vi "DFD Get Lattice Coef.vi"(7 "type (FLP)":enum16{"FLP", "FXP"}(ring), 8 "error in (no error)":errorcluster, 11 "filter in":T2={"mSRate_Fs"=1.0, "mSRate_Version"="2.0", "mSRate_Comments"="", "mSRate_OrgCoef"={"type"=enum."Undefined", "gain"=1.0, "coef a (k)"=[], "coef b (v)"=[]}, "mSRate_CurCoef"={"type"=enum."Undefined", "gain"=1.0, "coef a (k)"=[], "coef b (v)"=[]}, "mSRate_Quantized?"=FALSE, "mSRate_QCoef"={"type"=enum."Undefined", "gain"=1.0, "coef a (k)"=[], "coef b (v)"=[]}, "mSRate_QSettings"=[], "mSRate_Order"=0, "mSRate_Scaling"={"mSRate_ScaleByPowerOf2?"=FALSE, "mSRate_ScaleType"=enum."No Norm"}} {"mSRate_QSettings"."source" items=["Coef a/k"=0, "Coef b/v"=7, "Input"=1, "Output"=2, "Multiplicand"=3, "Product"=4, "Sum"=5, "Delay"=6, "Gain"=8]}) -> (0 "error out":errorcluster, 2 "lattice coef":T1 {"structure type" items=["Invalid"=0, "Lattice Allpass (basic sections)"=13, "Lattice Allpass (one multiplier sections)"=14, "Lattice Allpass (normalized sections)"=15, "Lattice AR (basic sections)"=16, "Lattice AR (one multiplier sections)"=17, "Lattice AR (normalized sections)"=18, "Lattice MA (minimum phase)"=19, "Lattice MA (maximum phase)"=20, "Lattice ARMA (basic sections)"=21, "Lattice ARMA (one multiplier sections)"=22, "Lattice ARMA (normalized sections)"=23]}, 3 "filter out":T2={"mSRate_Fs"=1.0, "mSRate_Version"="2.0", "mSRate_Comments"="", "mSRate_OrgCoef"={"type"=enum."Undefined", "gain"=1.0, "coef a (k)"=[], "coef b (v)"=[]}, "mSRate_CurCoef"={"type"=enum."Undefined", "gain"=1.0, "coef a (k)"=[], "coef b (v)"=[]}, "mSRate_Quantized?"=FALSE, "mSRate_QCoef"={"type"=enum."Undefined", "gain"=1.0, "coef a (k)"=[], "coef b (v)"=[]}, "mSRate_QSettings"=[], "mSRate_Order"=0, "mSRate_Scaling"={"mSRate_ScaleByPowerOf2?"=FALSE, "mSRate_ScaleType"=enum."No Norm"}} {"mSRate_QSettings"."source" items=["Coef a/k"=0, "Coef b/v"=7, "Input"=1, "Output"=2, "Multiplicand"=3, "Product"=4, "Sum"=5, "Delay"=6, "Gain"=8]})   [LabVIEW 2017, in "NI_DigFilterLicensed.lvlib"]
doc: "Retrieves the lattice form coefficients of a filter. The filter you specify must have a lattice form filter structure."
uses:
  <vilib>/addons/Digital Filter Design/NI_DigFilterLicensed.lvlib
  <vilib>/addons/Digital Filter Design/_Objects.llb/DFD Filter Obj.ctl
  <vilib>/addons/Digital Filter Design/_Objects.llb/DFD Filter Coef.ctl
  <vilib>/addons/Digital Filter Design/_Objects.llb/DFD Filter Structure Type Selector.ctl
  <vilib>/addons/Digital Filter Design/_Objects.llb/dfd_Internal Quantization Settings.ctl
  <vilib>/addons/Digital Filter Design/_Objects.llb/dfd_Internal Quantization Srcs.ctl
  <vilib>/addons/Digital Filter Design/_Objects.llb/DFD Coef Norm Type.ctl
  <vilib>/addons/Digital Filter Design/_Objects.llb/DFD Filter Structure Form Id.ctl
  <vilib>/addons/Digital Filter Design/_Misc.llb/dfd_Error Cluster From Error Code (Scalar).vi
  <vilib>/addons/Digital Filter Design/FilterLib.llb/dfd_Get Filter Coef Type (Filter IO).vi
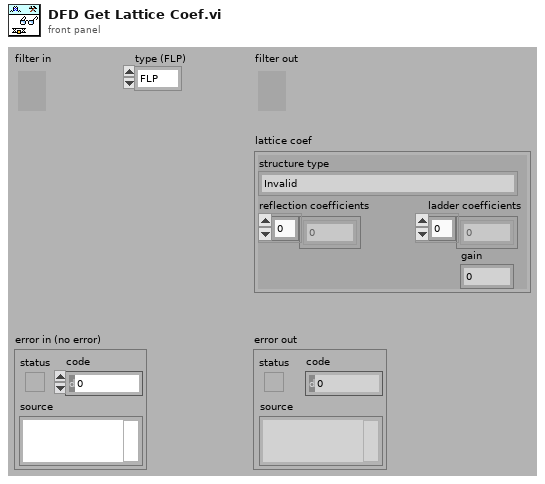
[diagram p1: front panel]
types:
  T1 = cluster{"structure type":u16, "reflection coefficients":dbl[], "ladder coefficients":dbl[], "gain":dbl}
  T2 = typedef "NI_DigFilterLicensed.lvlib/DFD Filter Obj.ctl" = cluster{"mSRate_Fs":dbl, "mSRate_Version":string, "mSRate_Comments":string, "mSRate_OrgCoef":T3, "mSRate_CurCoef":T3, "mSRate_Quantized?":bool, "mSRate_QCoef":T3, "mSRate_QSettings":T5[], "mSRate_Order":i32, "mSRate_Scaling":cluster{"mSRate_ScaleByPowerOf2?":bool, "mSRate_ScaleType":T7}}
  T3 = typedef "NI_DigFilterLicensed.lvlib/DFD Filter Coef.ctl" = cluster{"type":T4, "gain":dbl, "coef a (k)":dbl[], "coef b (v)":dbl[]}
  T4 = typedef "NI_DigFilterLicensed.lvlib/DFD Filter Structure Type Selector.ctl" = enum16{"Undefined", "FIR Direct Form", "FIR Direct Form Transposed", "FIR Symmetric", "FIR Antisymmetric", "IIR Direct Form I", "IIR Direct Form I Transposed", "IIR Direct Form II", "IIR Direct Form II Transposed", "IIR Cascaded Second Order Sections Form I", "IIR Cascaded Second Order Sections Form I Transposed", "IIR Cascaded Second Order Sections Form II", "IIR Cascaded Second Order Sections Form II Transposed", "Lattice Allpass (basic sections)", "Lattice Allpass (one multiplier sections)", "Lattice Allpass (normalized sections)", "Lattice AR (basic sections)", "Lattice AR (one multiplier sections)", "Lattice AR (normalized sections)", "Lattice MA (minimum phase)", "Lattice MA (maximum phase)", "Lattice ARMA (basic sections)", "Lattice ARMA (one multiplier sections)", "Lattice ARMA (normalized sections)"}
  T5 = typedef "NI_DigFilterLicensed.lvlib/dfd_Internal Quantization Settings.ctl" = cluster{"source":T6, "wl":i16, "iwl":i16, "overflow mode":enum16{"Saturation", "Wrap"}, "rounding mode":enum16{"Nearest", "Truncation"}, "signed?":bool}
  T6 = typedef "NI_DigFilterLicensed.lvlib/dfd_Internal Quantization Srcs.ctl" = u16
  T7 = typedef "NI_DigFilterLicensed.lvlib/DFD Coef Norm Type.ctl" = enum16{"No Norm", "Time Domain 1-Norm", "Time Domain 2-Norm", "Time Domain Inf-Norm"}
  T8 = typedef "NI_DigFilterLicensed.lvlib/DFD Filter Structure Form Id.ctl" = enum16{"Undefined", "Direct Form", "SOS Form", "Lattice Form"}
  T9 = cluster{"structure type":T4, "k":dbl[], "v":dbl[], "gain":dbl}
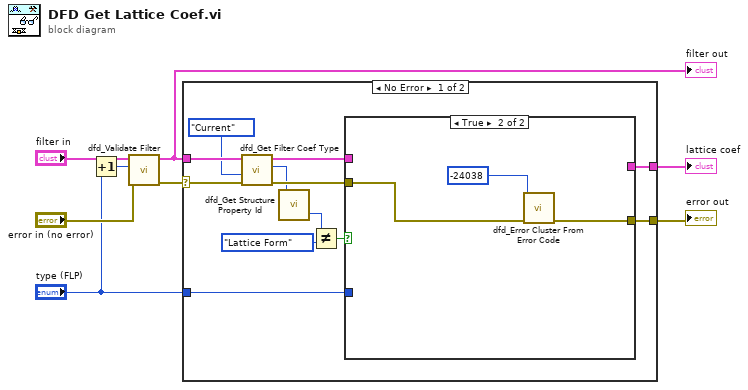
[diagram p0: block diagram]
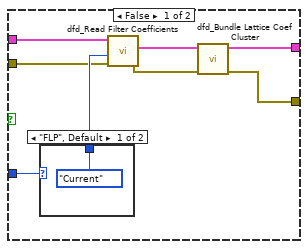
[diagram p2: hidden frame]
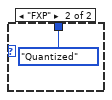
[diagram p3: hidden frame]
diagram:
  n1 = Increment(x="type (FLP)") -> (x+1=w2:enum16{"FLP", "FXP"})
  n2 = call <vilib>:"dfd_Validate Filter.vi"("error in (no error)"="error in (no error)", "check option"=w2, "filter in"="filter in") -> ("error out"=w3:errorcluster, "filter out"=w5:T2)  [unwired: 7 out]
  "filter out" <- w5
  n3 = case shown="No Error" w3 {
    selector: w3 -> [w12 w34]
    tunnel: [w16 w34] -> w8
    tunnel: w5 -> [w14 _]
    tunnel: [w17 _] -> w7
    tunnel: "type (FLP)" -> [w15 _]
    frame No Error {
      n4 = call-poly <vilib>:"dfd_Get Filter Coef Type.vi"("error in (no error)"=w12, "coef source"=enum16{"Original", "Current", "Quantized"}."Current", "filter in"=w14) -> ("error out"=w10:errorcluster, "type"=w9:T4, "filter out"=w13:T2)  [unwired: 1 in, 5 out]
      n5 = call <vilib>:"dfd_Get Structure Property Id.vi"("structure type"=w9) -> ("filter structure form id"=w19:T8)  [unwired: 1 out]
      n6 = Not Equal?(x=w19, y=DFD_Filter_Structure_Form_Id."Lattice Form" ("filter structure form id")) -> (x != y?=w18:bool)
      n7 = case shown="True" w18 {
        tunnel: w13 -> [w28 _]
        tunnel: [w25 _] -> w17
        tunnel: [w24 w32] -> w16
        tunnel: w15 -> [w23 _]
        tunnel: w10 -> [w21 w31]
        frame False {
          n8 = case shown="\"FLP\", Default" w23 {
            tunnel: [enum16{"Original", "Current", "Quantized"}."Current" ("coef source") enum16{"Original", "Current", "Quantized"}."Quantized" ("coef source")] -> w22
            frame "FLP", Default {
            }
            frame "FXP" {
            }
          }
          n9 = call <vilib>:"dfd_Read Filter Coefficients.vi"("error in (no error)"=w21, "coef source"=w22, "filter in"=w28) -> ("error out"=w26:errorcluster, "filter coef"=w27:T3)  [unwired: 7 out]
          n10 = call <vilib>:"dfd_Bundle Lattice Coef Cluster.vi"("error in (no error)"=w26, "filter coef"=w27) -> ("error out"=w24:errorcluster, "lattice coef"=w25:T9)  [unwired: 1 in, 7 out]
        }
        frame True {
          n11 = call-poly <vilib>:"dfd_Error Cluster From Error Code.vi"("error in (no error)"=w31, "error code (0)"=-24038 ("ERR_NOT_LATTICE_COEF")) -> ("error out"=w32:errorcluster)  [unwired: 9 out]
        }
      }
    }
    frame Error {
    }
  }
  "error out" <- w8
  "lattice coef" <- w7
